vi "configcode.vi"(0 "object in":refnum<class "interface.lvclass">, 5 "error in (no error)":errorcluster) -> (14 "object out":refnum<class "interface.lvclass">, 19 "error out":errorcluster)   [LabVIEW 2016, in "interface.lvclass"]
uses:
  interface.lvclass
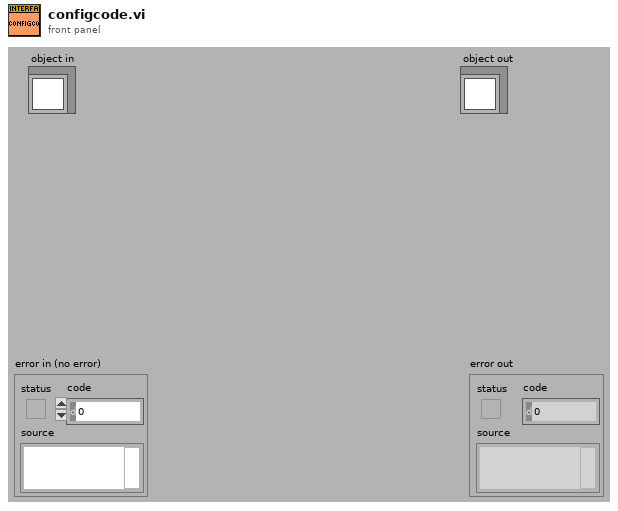
[diagram p1: front panel]
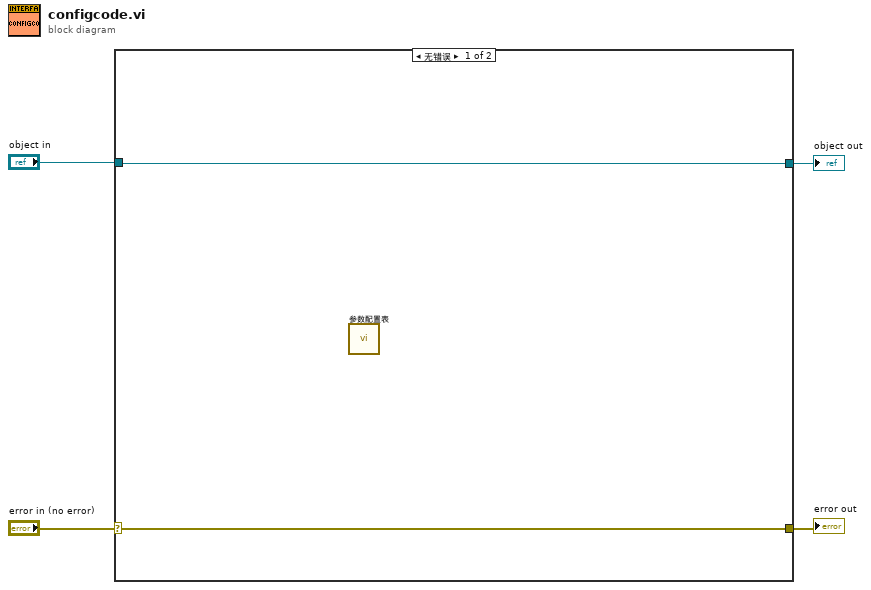
[diagram p0: block diagram]
diagram:
  n1 = case shown="无错误" "error in (no error)" {
    selector: "error in (no error)" -> [w6 w8]
    tunnel: [w6 w8] -> w3
    tunnel: [w5 w7] -> w1
    tunnel: "object in" -> [w5 w7]
    frame No Error {
      n2 = call "参数配置表.vi"() -> ()  [unwired: 12 in]
    }
    frame Error {
    }
  }
  "error out" <- w3
  "object out" <- w1
